vi "Function.vi"(8 "error in (no error)":errorcluster, 9 "B":T1, 10 "A":T1, 11 "NOR in":refnum<class "NOR_U16.lvclass">) -> (0 "error out":errorcluster, 2 "Result":T1, 3 "NOR out":refnum<class "NOR_U16.lvclass">)   [LabVIEW 2021, in "NOR_U16.lvclass"]
uses:
  NOR_U16.lvclass
  Type.ctl
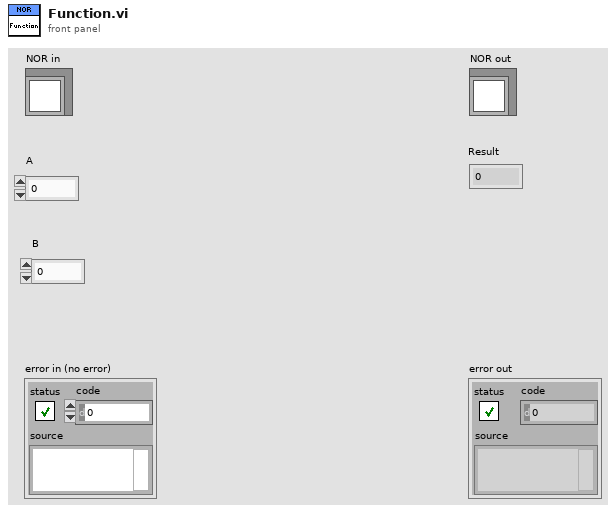
[diagram p1: front panel]
types:
  T1 = typedef "NOR_U16.lvclass/Type.ctl" = u16
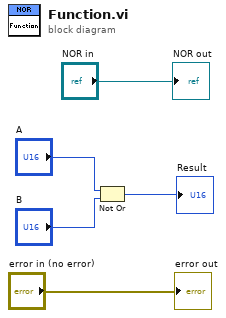
[diagram p0: block diagram]
diagram:
  n1 = Not Or(1:"B", 2:"A") -> (0:→"Result":T1)
  "error out" <- "error in (no error)"
  "NOR out" <- "NOR in"
